vi "Controller - State Entry.vi"(8 "error in (no error)":errorcluster, 11 "View Model":T1) -> (0 "error out":errorcluster, 3 "View Model":T1)   [LabVIEW 2017]
doc: "Orginize state transition and process Entry new state"
uses:
  View Model/Controls/View Model.ctl
  Configuration Database/Controls/Config Model.ctl
  Configuration Database/Controls/Config Commands.ctl
  Configuration Database/Controls/Congif Data.ctl
  View Model/Controls/Shared Model.ctl
  Error Handler/Controls/Error Model.ctl
  Error Handler/Controls/Error Data.ctl
  Error Handler/Controls/Error Type.ctl
  Controls/Car Wash Model.ctl
  Controls/Controller Overhead.ctl
  Controls/Vehicle Location.ctl
  Controls/Car Wash States.ctl
  Controls/CarWash CMD.ctl
  Views/Wash Display Console View/Controls/Car Wash Indicators.ctl
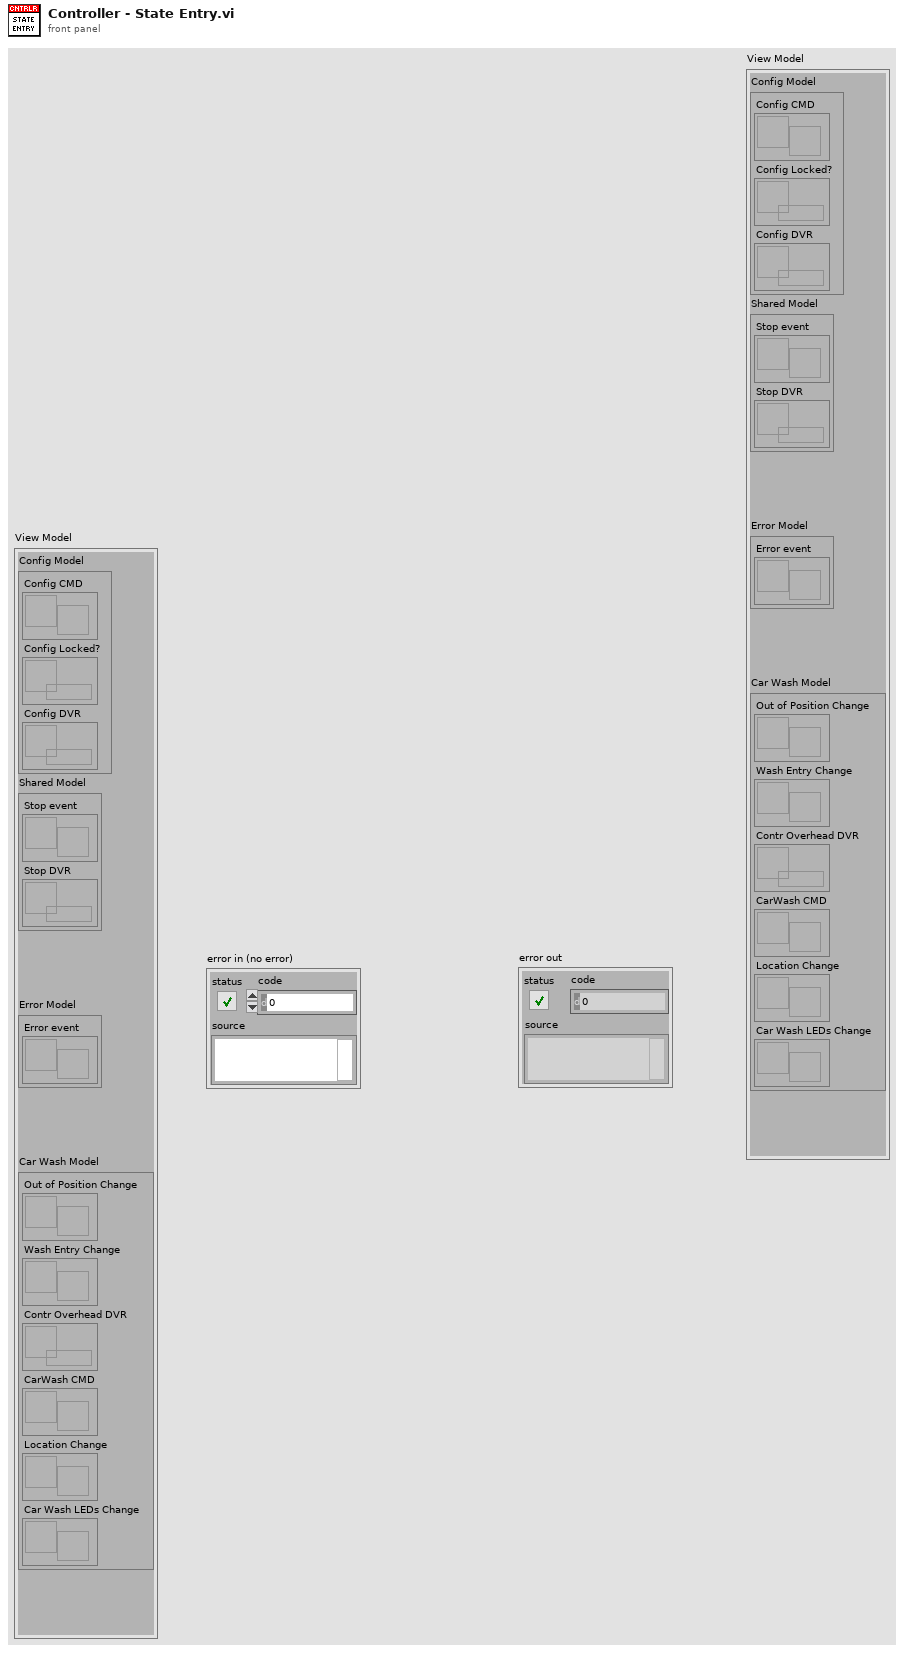
[diagram p1: front panel]
types:
  T1 = typedef "View Model.ctl" = cluster{"Config Model":T2, "Shared Model":T3, "Error Model":T4, "Car Wash Model":T5}
  T2 = typedef "Config Model.ctl" = cluster{"Config CMD":refnum<user-event>, "Config Locked?":refnum<data-value>, "Config DVR":refnum<data-value>}
  T3 = typedef "Shared Model.ctl" = cluster{"Stop event":refnum<user-event>, "Stop DVR":refnum<data-value>}
  T4 = typedef "Error Model.ctl" = cluster{"Error event":refnum<user-event>}
  T5 = typedef "Car Wash Model.ctl" = cluster{"Out of Position Change":refnum<user-event>, "Wash Entry Change":refnum<user-event>, "Contr Overhead DVR":refnum<data-value>, "CarWash CMD":refnum<user-event>, "Location Change":refnum<user-event>, "Car Wash LEDs Change":refnum<user-event>}
  T6 = typedef "Car Wash States.ctl" = enum16{"Initial", "Wait for start", "Start", "Wait for vehicle", "Wash Step Execution", "Wash Step/Cycle Complete", "Wash Exit", "Wash Abort/Terminate"}
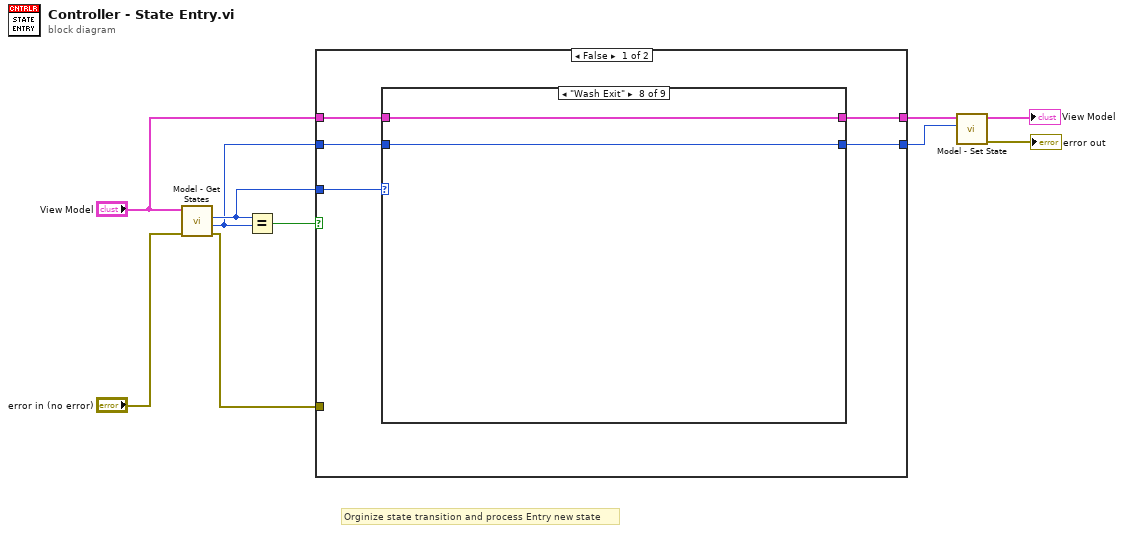
[diagram p0: block diagram]
diagram:
  # "Orginize state transition and process Entry new state"
  n1 = call "Model - Get States.vi"("error in (no error)"="error in (no error)", "View Model"="View Model") -> ("error out"=w1:errorcluster, "CarWash Next State"=w7:T6, "CarWash State"=w8:T6)  [unwired: 6 in, 1 out]
  n2 = Equal?(x=w8, y=w7) -> (x = y?=w9:bool)
  n3 = case shown="False" w9 {
    tunnel: w8 -> [w15 _]
    tunnel: w7 -> [w12 w34]
    tunnel: "View Model" -> [w14 w35]
    tunnel: [w13 w35] -> w5
    tunnel: [w11 w34] -> w4
    tunnel: w1 -> [_ _]
    frame False {
      n4 = case shown="\"Wash Exit\"" w15 {
        tunnel: w14 -> [w17 w19 w21 w23 w25 w27 w29 w31 w33]
        tunnel: [w17 w19 w21 w23 w25 w27 w29 w31 w33] -> w13
        tunnel: w12 -> [w16 w18 w20 w22 w24 w26 w28 w30 w32]
        tunnel: [w16 w18 w20 w22 w24 w26 w28 w30 w32] -> w11
        frame Default {
        }
        frame "Initial" {
        }
        frame "Wait for start" {
          # "[Covers: WS1]"
          # "#TODO\n- Maintain Initial State Requirements"
        }
        frame "Start" {
          # "[Covers: SS1]"
          # "#TODO\n- Disable the Entry Console controls"
        }
        frame "Wait for vehicle" {
        }
        frame "Wash Step Execution" {
          # "[Covers: WX1]"
          # "#TODO\n- Wait the correct car position on the appropriate station"
        }
        frame "Wash Step/Cycle Complete" {
        }
        frame "Wash Exit" {
        }
        frame "Wash Abort/Terminate" {
        }
      }
    }
    frame True {
    }
  }
  n5 = call "Model - Set State.vi"("CarWash Next State"=w4, "View Model"=w5) -> ("error out"=→"error out":errorcluster, "View Model"=→"View Model":T1)  [unwired: 8 in]
